vi "Constructor.vi"(8 "error in (no error)":errorcluster, 11 "Module Settings":T1) -> (0 "error out":errorcluster, 2 "Use?":bool, 3 "Module.lvclass":refnum<class "Module.lvclass">)   [LabVIEW 2025, in "Module.lvclass"]
doc: "Instantiate specific module class with configured signals."
uses:
  Module.lvclass
  Module Settings.ctl
  Signal/Signal/Signal Settings.ctl
  Input Module/Input Module.lvclass
  C:/Projects/VeriStand-FPGA-Generation-Wizard/Source/Classes/Module/Module/Module.lvclass
  Output Module/Output Module.lvclass
  VI/VI/Error Codes.ctl
  Module.lvclass/Module.ctl
  Signal/Signal/Signal.lvclass
  VI/VI/VI.lvclass
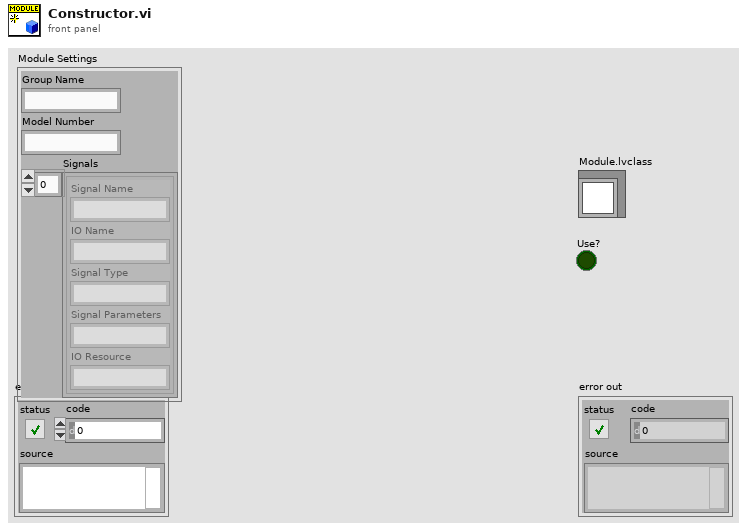
[diagram p1: front panel]
types:
  T1 = typedef "Module.lvclass/Module Settings.ctl" = cluster{"Group Name":string, "Model Number":string, "Signals":T2[]}
  T2 = typedef "Signal.lvclass/Signal Settings.ctl" = cluster{"Signal Name":string, "IO Name":string, "Signal Type":string, "Signal Parameters":string, "IO Resource":string}
  T3 = typedef "VI.lvclass/Error Codes.ctl" = enum16{"Signal Unsupported", "Module Unsupported", "Parameter Unsupported", "Signal Code Gen Error", "Module Code Gen Error", "Cleanup Code Error", "Signal Direction Mismatch", "Signal Type Mismatch", "Module Channel Number Mismatch", "Minimum Channels Mismatch"}
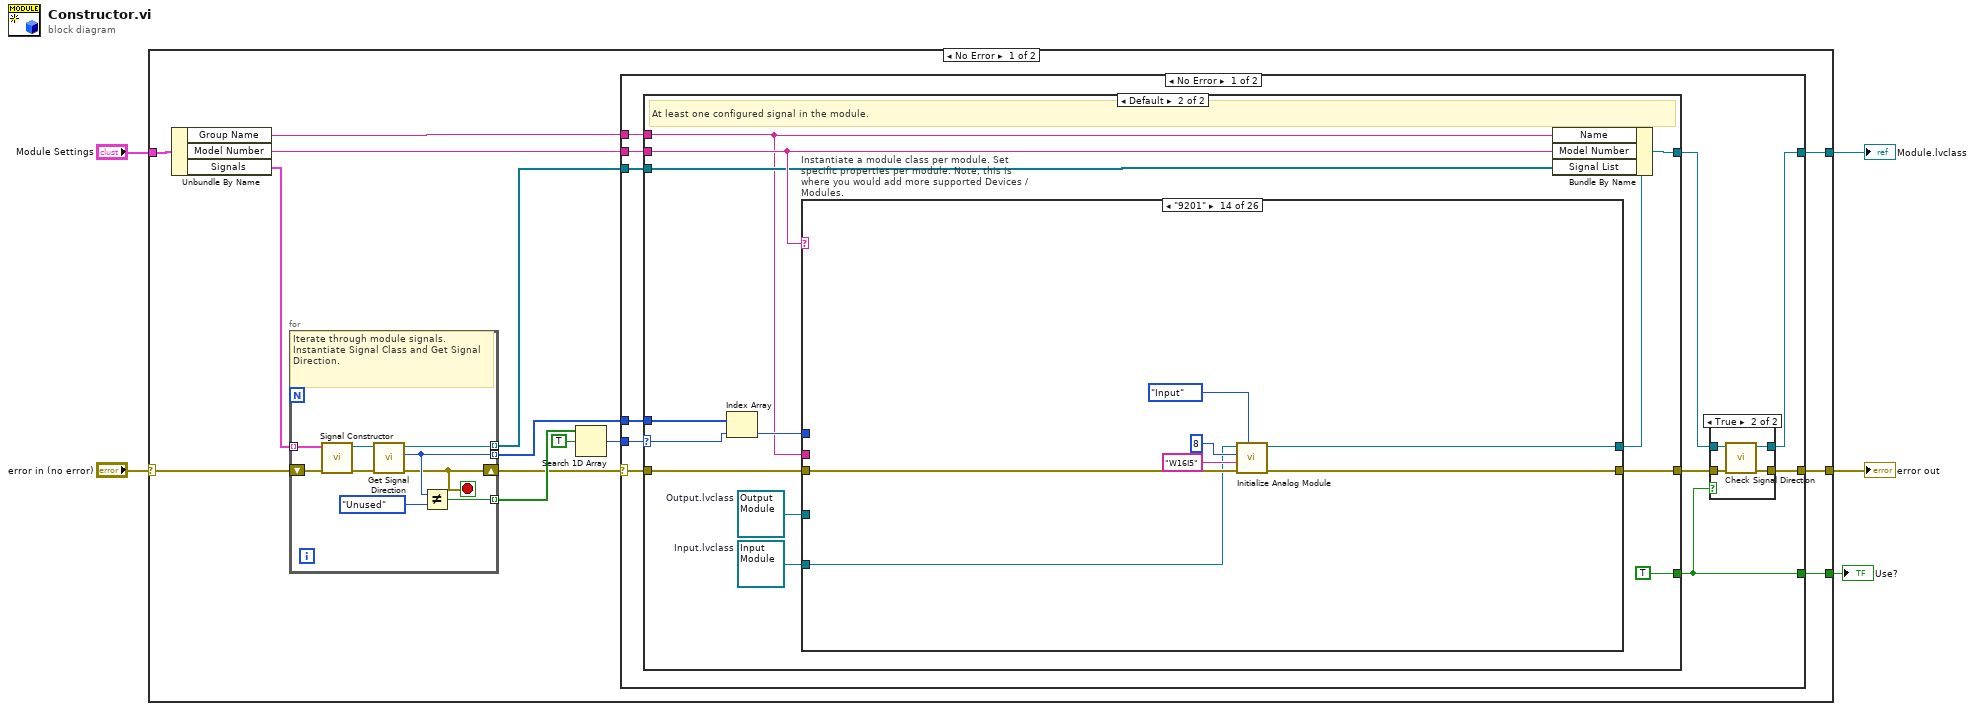
[diagram p0: block diagram]
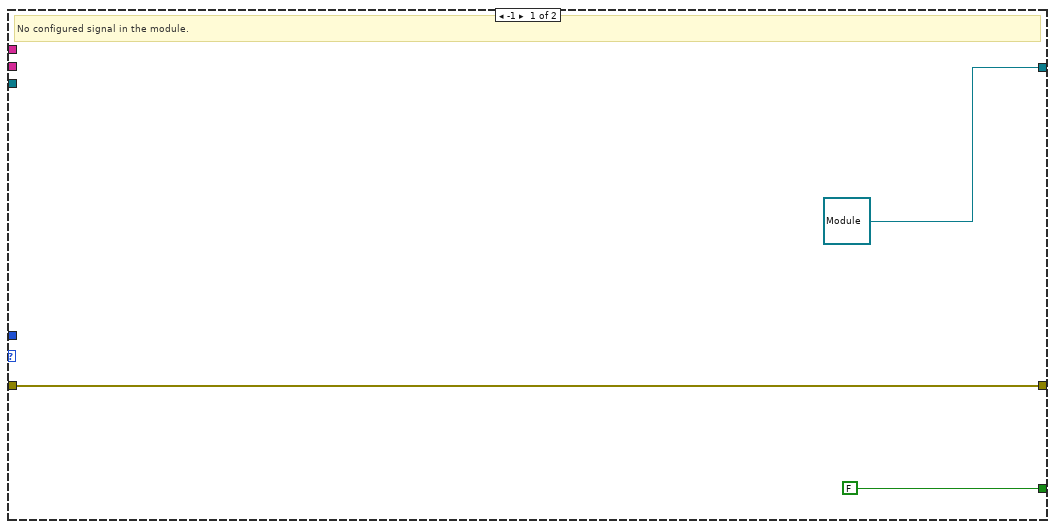
[diagram p3: hidden frame]
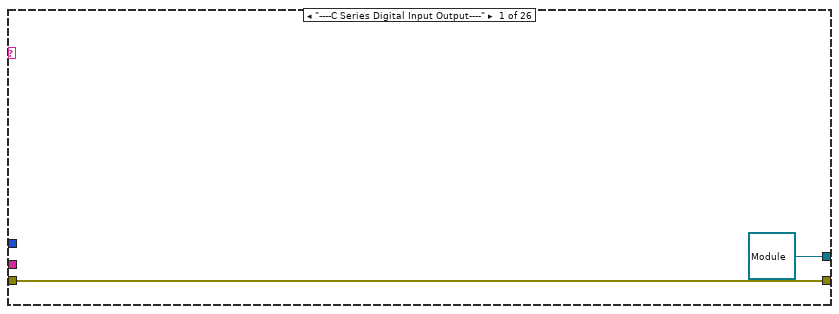
[diagram p4: hidden frame]
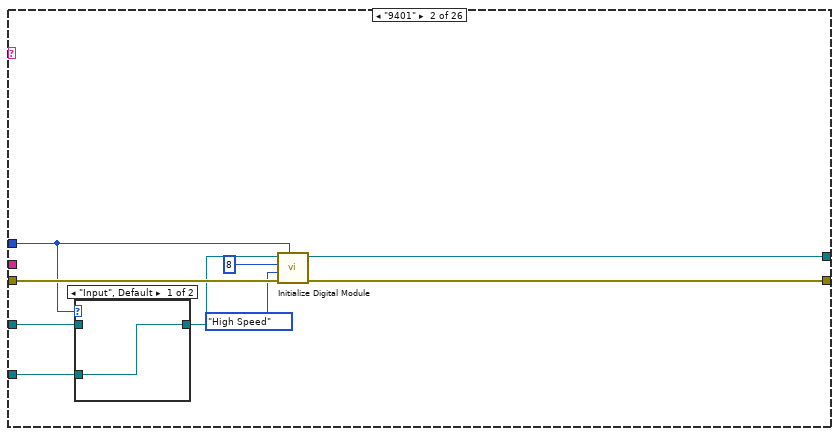
[diagram p5: hidden frame]
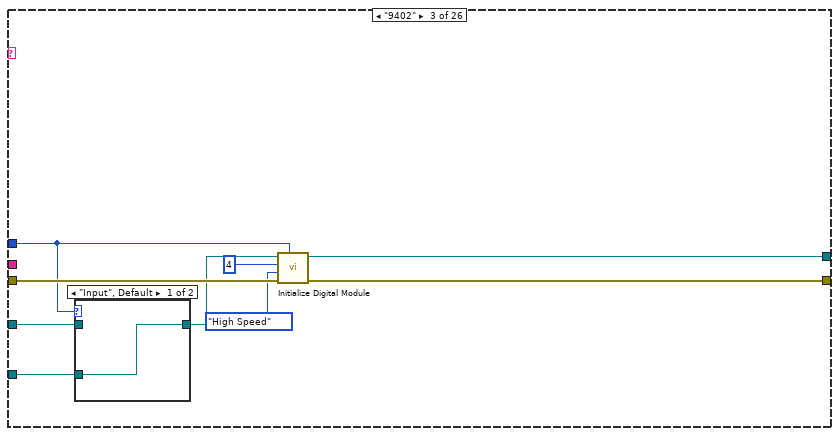
[diagram p7: hidden frame]
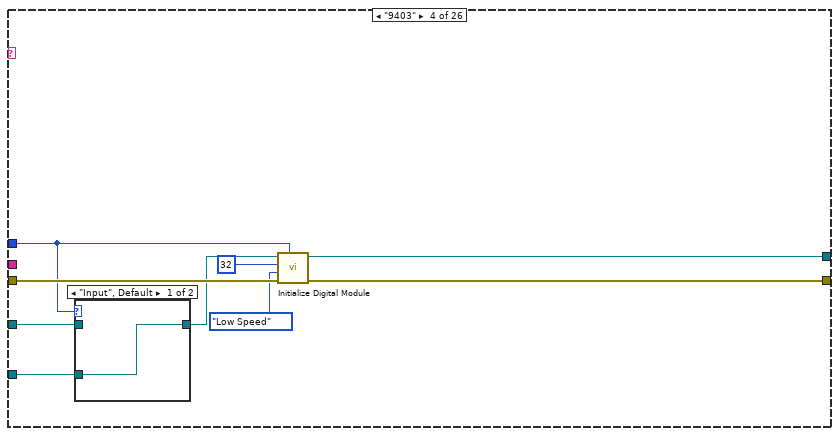
[diagram p9: hidden frame]
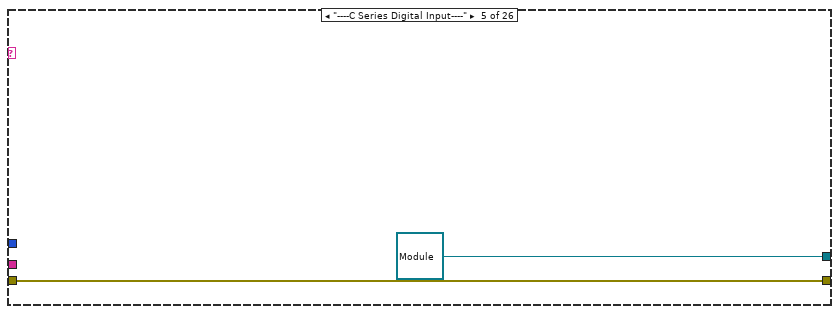
[diagram p11: hidden frame]
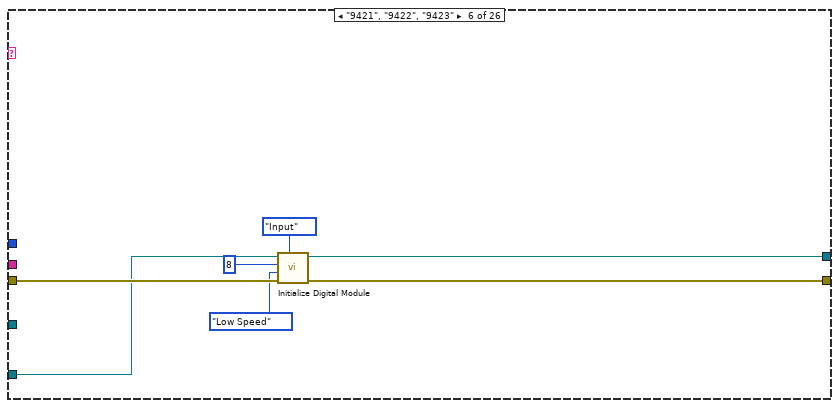
[diagram p12: hidden frame]
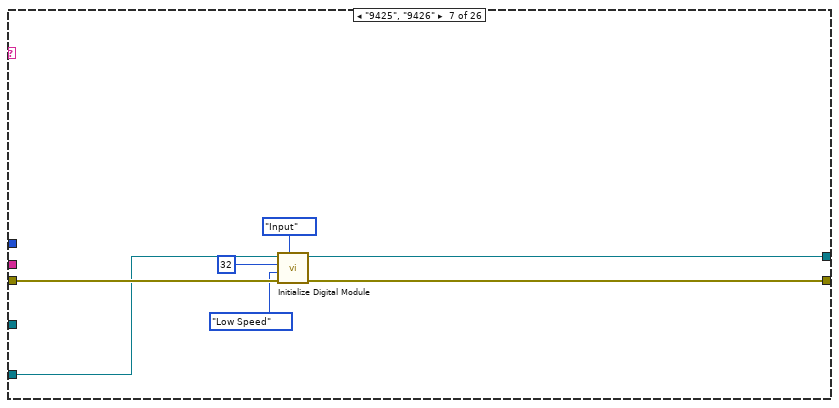
[diagram p13: hidden frame]
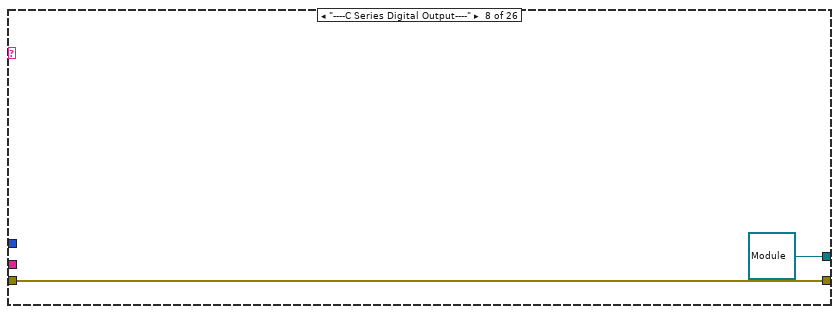
[diagram p14: hidden frame]
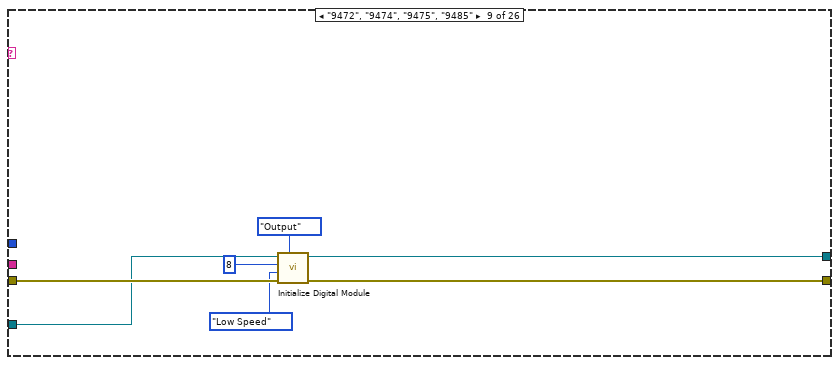
[diagram p15: hidden frame]
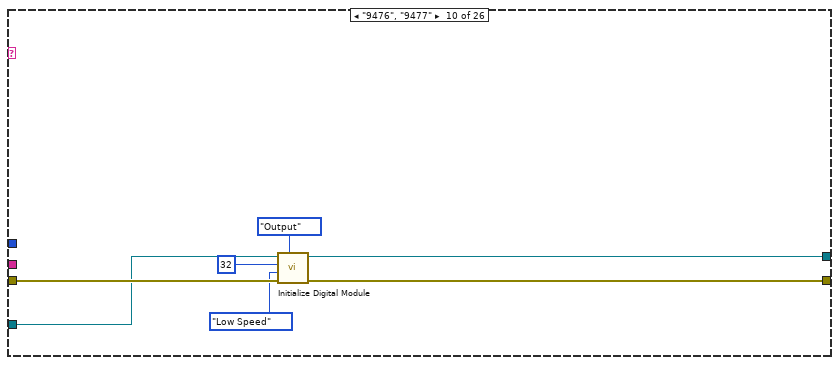
[diagram p16: hidden frame]
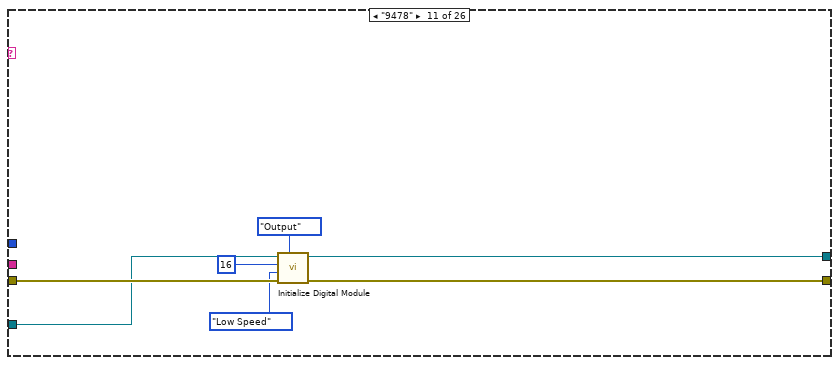
[diagram p17: hidden frame]
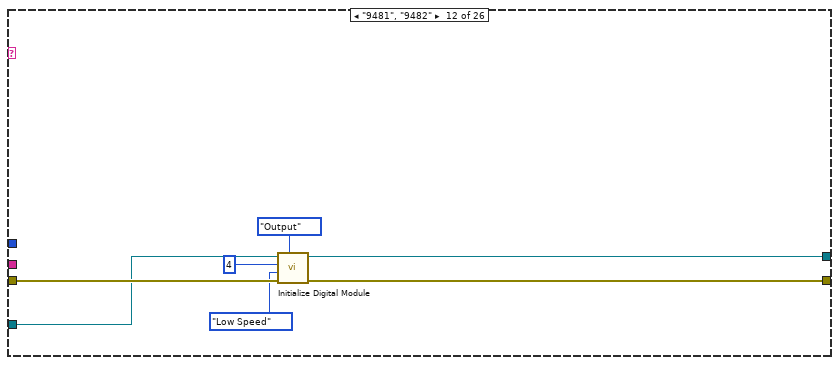
[diagram p18: hidden frame]
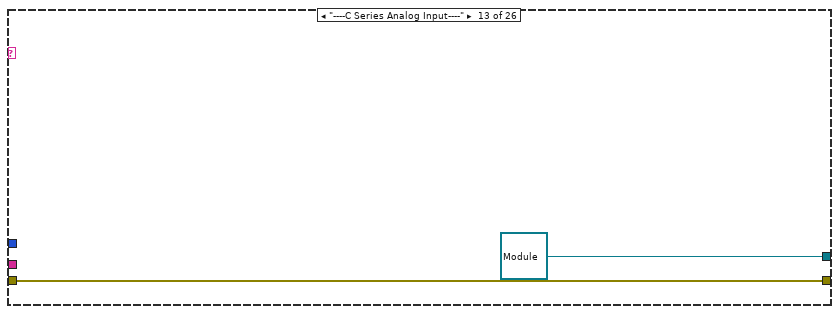
[diagram p19: hidden frame]
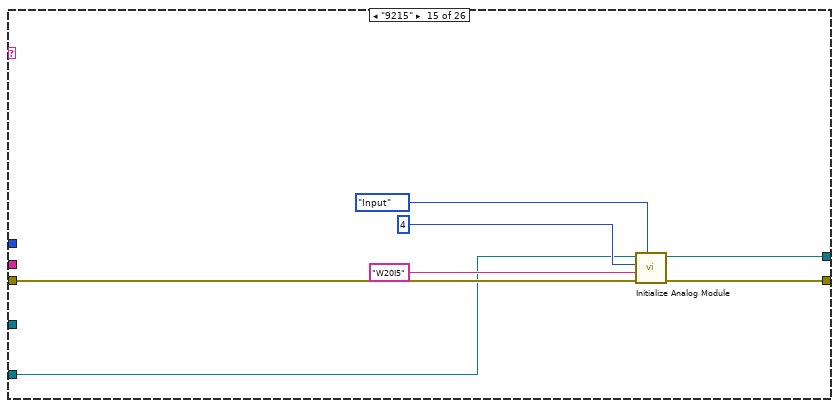
[diagram p20: hidden frame]
diagram:
  n1 = case shown="No Error" "error in (no error)" {
    selector: "error in (no error)" -> [w13 w285]
    tunnel: "Module Settings" -> [w19 _]
    tunnel: [w18 refnum<class "Module.lvclass"> refnum ("Module out")] -> w4
    tunnel: [w15 w285] -> w2
    tunnel: [w7 FALSE] -> w1
    frame No Error {
      n2 = Unbundle By Name(w19) -> ("Group Name"=w17:string, "Model Number"=w16:string, "Signals"=w14:T2[])
      n3 = for {
        tunnel: w14 -> [w282] mode=indexing
        shift-right: [w274] -> w6
        shift-left: w13 -> [w281]
        tunnel: [w278] -> w12 mode=indexing
        tunnel: [w277] -> w9 mode=indexing
        tunnel: [w275] -> w11 mode=indexing
        stop <- w274 stop-if-true
        # "Iterate through module signals. Instantiate Signal Class and Get Signal Direction."
        n4 = call "Signal Constructor.vi"("error in (no error)"=w281, "Signal Settings"=w282) -> ("error out"=w280:errorcluster, "IO Class.lvclass"=w279:refnum<class "Signal.lvclass">)  [unwired: 8 in]
        n5 = call "Get Signal Direction.vi"("error in (no error)"=w280, "IO Class in"=w279) -> ("error out"=w274:errorcluster, "Direction"=w277:enum16{"Input", "Output", "Unused"}, "IO Class out"=w278:refnum<class "Signal.lvclass">)  [unwired: 7 in]
        n6 = Not Equal?(x=w277, y=enum16{"Input", "Output", "Unused"}."Unused" ("Direction")) -> (x != y?=w275:bool)
      }
      n7 = Search 1D Array(1D array=w11, element=TRUE) -> (index of element=w8:i32)  [unwired: 1 in]
      n8 = case shown="No Error" w6 {
        selector: w6 -> [w25 w273]
        tunnel: [w21 refnum<class "Module.lvclass"> refnum ("Module out")] -> w18
        tunnel: w17 -> [w30 _]
        tunnel: w16 -> [w29 _]
        tunnel: [w23 w273] -> w15
        tunnel: w12 -> [w28 _]
        tunnel: w9 -> [w27 _]
        tunnel: w8 -> [w26 _]
        tunnel: [w20 _] -> w7
        frame No Error {
          n9 = case shown="Default" w26 {
            selector: w26 -> [_ w42]
            tunnel: [refnum<class "Module.lvclass"> refnum ("Module out") w51] -> w22
            tunnel: w30 -> [_ w40]
            tunnel: w29 -> [_ w50]
            tunnel: [w39 w49] -> w24
            tunnel: w28 -> [_ w46]
            tunnel: w25 -> [w39 w45]
            tunnel: w27 -> [_ w44]
            tunnel: [FALSE TRUE] -> w20
            frame -1 {
              # "No configured signal in the module."
            }
            frame Default {
              w47 = refnum<class "Output Module.lvclass"> refnum  # Output.lvclass
              w48 = refnum<class "Input Module.lvclass"> refnum  # Input.lvclass
              # "At least one configured signal in the module."
              n10 = Index Array(array=w44, index=w42) -> (element=w43:enum16{"Input", "Output", "Unused"})
              n11 = case "Instantiate a module class per module. Set specific properties per module. Note, this is where you would add more supported Devices / Modules." shown="\"9201\"" w50 {
                selector: w50 -> [_ _ _ _ _ _ _ _ _ _ _ _ _ _ _ _ _ _ _ _ _ _ _ _ _ w210]
                tunnel: [refnum<class "Module.lvclass"> refnum ("Module out") w63 w74 w85 refnum<class "Module.lvclass"> refnum ("Module out") w96 w103 refnum<class "Module.lvclass"> refnum ("Module out") w112 w119 w126 w133 refnum<class "Module.lvclass"> refnum ("Module out") w142 w149 w156 w163 w170 w177 w184 refnum<class "Module.lvclass"> refnum ("Module out") w193 w200 w207 refnum<class "Module.lvclass"> refnum ("Module out") w216] -> w52
                tunnel: w45 -> [w54 w62 w73 w84 w89 w95 w102 w105 w111 w118 w125 w132 w135 w137 w144 w151 w158 w165 w172 w179 w186 w192 w199 w206 w209 w220]
                tunnel: [w54 w61 w72 w83 w89 w94 w101 w105 w110 w117 w124 w131 w135 w141 w148 w155 w162 w169 w176 w183 w186 w191 w198 w205 w209 w215] -> w49
                tunnel: w43 -> [_ w58 w69 w80 _ _ _ _ _ _ _ _ _ _ _ _ _ _ _ _ _ _ _ _ _ w217]
                tunnel: w48 -> [_ w56 w67 w78 _ w91 w98 _ _ _ _ _ _ w136 w143 w150 w157 w164 w171 w178 _ _ _ _ _ w218]
                tunnel: w47 -> [_ w57 w68 w79 _ _ _ _ w106 w113 w120 w127 _ _ _ _ _ _ _ _ _ w187 w194 w201 _ w219]
                tunnel: w40 -> [_ _ _ _ _ _ _ _ _ _ _ _ _ _ _ _ _ _ _ _ _ _ _ _ _ w221]
                frame "----C Series Digital Input Output----" {
                }
                frame "9401" {
                  n12 = case shown="\"Input\", Default" w58 {
                    tunnel: w57 -> [_ w65]
                    tunnel: w56 -> [w64 _]
                    tunnel: [w64 w65] -> w55
                    frame "Input", Default {
                    }
                    frame "Output" {
                    }
                  }
                  n13 = call "Initialize Digital Module.vi"("Direction"=w58, "error in (no error)"=w62, "Speed"=enum16{"High Speed", "Low Speed"}."High Speed", "Channels"=u8 8, "Module in"=w55) -> ("error out"=w61:errorcluster, "Module out"=w63:refnum<class "Module.lvclass">)  [unwired: 5 in]
                }
                frame "9402" {
                  n14 = case shown="\"Input\", Default" w69 {
                    tunnel: w68 -> [_ w76]
                    tunnel: w67 -> [w75 _]
                    tunnel: [w75 w76] -> w66
                    frame "Input", Default {
                    }
                    frame "Output" {
                    }
                  }
                  n15 = call "Initialize Digital Module.vi"("Direction"=w69, "error in (no error)"=w73, "Speed"=enum16{"High Speed", "Low Speed"}."High Speed", "Channels"=u8 4, "Module in"=w66) -> ("error out"=w72:errorcluster, "Module out"=w74:refnum<class "Module.lvclass">)  [unwired: 5 in]
                }
                frame "9403" {
                  n16 = case shown="\"Input\", Default" w80 {
                    tunnel: w79 -> [_ w87]
                    tunnel: w78 -> [w86 _]
                    tunnel: [w86 w87] -> w77
                    frame "Input", Default {
                    }
                    frame "Output" {
                    }
                  }
                  n17 = call "Initialize Digital Module.vi"("Direction"=w80, "error in (no error)"=w84, "Speed"=enum16{"High Speed", "Low Speed"}."Low Speed", "Channels"=u8 32, "Module in"=w77) -> ("error out"=w83:errorcluster, "Module out"=w85:refnum<class "Module.lvclass">)  [unwired: 5 in]
                }
                frame "----C Series Digital Input----" {
                }
                frame "9421", "9422", "9423" {
                  n18 = call "Initialize Digital Module.vi"("Direction"=enum16{"Input", "Output"}."Input", "error in (no error)"=w95, "Speed"=enum16{"High Speed", "Low Speed"}."Low Speed", "Channels"=u8 8, "Module in"=w91) -> ("error out"=w94:errorcluster, "Module out"=w96:refnum<class "Input Module.lvclass">)  [unwired: 5 in]
                }
                frame "9425", "9426" {
                  n19 = call "Initialize Digital Module.vi"("Direction"=enum16{"Input", "Output"}."Input", "error in (no error)"=w102, "Speed"=enum16{"High Speed", "Low Speed"}."Low Speed", "Channels"=u8 32, "Module in"=w98) -> ("error out"=w101:errorcluster, "Module out"=w103:refnum<class "Input Module.lvclass">)  [unwired: 5 in]
                }
                frame "----C Series Digital Output----" {
                }
                frame "9472", "9474", "9475", "9485" {
                  n20 = call "Initialize Digital Module.vi"("Direction"=enum16{"Input", "Output"}."Output", "error in (no error)"=w111, "Speed"=enum16{"High Speed", "Low Speed"}."Low Speed", "Channels"=u8 8, "Module in"=w106) -> ("error out"=w110:errorcluster, "Module out"=w112:refnum<class "Output Module.lvclass">)  [unwired: 5 in]
                }
                frame "9476", "9477" {
                  n21 = call "Initialize Digital Module.vi"("Direction"=enum16{"Input", "Output"}."Output", "error in (no error)"=w118, "Speed"=enum16{"High Speed", "Low Speed"}."Low Speed", "Channels"=u8 32, "Module in"=w113) -> ("error out"=w117:errorcluster, "Module out"=w119:refnum<class "Output Module.lvclass">)  [unwired: 5 in]
                }
                frame "9478" {
                  n22 = call "Initialize Digital Module.vi"("Direction"=enum16{"Input", "Output"}."Output", "error in (no error)"=w125, "Speed"=enum16{"High Speed", "Low Speed"}."Low Speed", "Channels"=u8 16, "Module in"=w120) -> ("error out"=w124:errorcluster, "Module out"=w126:refnum<class "Output Module.lvclass">)  [unwired: 5 in]
                }
                frame "9481", "9482" {
                  n23 = call "Initialize Digital Module.vi"("Direction"=enum16{"Input", "Output"}."Output", "error in (no error)"=w132, "Speed"=enum16{"High Speed", "Low Speed"}."Low Speed", "Channels"=u8 4, "Module in"=w127) -> ("error out"=w131:errorcluster, "Module out"=w133:refnum<class "Output Module.lvclass">)  [unwired: 5 in]
                }
                frame "----C Series Analog Input----" {
                }
                frame "9201" {
                  n24 = call "Initialize Analog Module.vi"("Direction"=enum16{"Input", "Output"}."Input", "error in (no error)"=w137, "FXP Type"="W16I5", "Channels"=u8 8, "Module in"=w136) -> ("error out"=w141:errorcluster, "Module out"=w142:refnum<class "Input Module.lvclass">)  [unwired: 5 in]
                }
                frame "9215" {
                  n25 = call "Initialize Analog Module.vi"("Direction"=enum16{"Input", "Output"}."Input", "error in (no error)"=w144, "FXP Type"="W20I5", "Channels"=u8 4, "Module in"=w143) -> ("error out"=w148:errorcluster, "Module out"=w149:refnum<class "Input Module.lvclass">)  [unwired: 5 in]
                }
                frame "9220" {
                  n26 = call "Initialize Analog Module.vi"("Direction"=enum16{"Input", "Output"}."Input", "error in (no error)"=w151, "FXP Type"="W24I5", "Channels"=u8 16, "Module in"=w150) -> ("error out"=w155:errorcluster, "Module out"=w156:refnum<class "Input Module.lvclass">)  [unwired: 5 in]
                }
                frame "9221" {
                  n27 = call "Initialize Analog Module.vi"("Direction"=enum16{"Input", "Output"}."Input", "error in (no error)"=w158, "FXP Type"="W16I7", "Channels"=u8 8, "Module in"=w157) -> ("error out"=w162:errorcluster, "Module out"=w163:refnum<class "Input Module.lvclass">)  [unwired: 5 in]
                }
                frame "9222", "9223" {
                  n28 = call "Initialize Analog Module.vi"("Direction"=enum16{"Input", "Output"}."Input", "error in (no error)"=w165, "FXP Type"="W24I5", "Channels"=u8 4, "Module in"=w164) -> ("error out"=w169:errorcluster, "Module out"=w170:refnum<class "Input Module.lvclass">)  [unwired: 5 in]
                }
                frame "9224" {
                  n29 = call "Initialize Analog Module.vi"("Direction"=enum16{"Input", "Output"}."Input", "error in (no error)"=w172, "FXP Type"="W24I5", "Channels"=u8 8, "Module in"=w171) -> ("error out"=w176:errorcluster, "Module out"=w177:refnum<class "Input Module.lvclass">)  [unwired: 5 in]
                }
                frame "9228" {
                  n30 = call "Initialize Analog Module.vi"("Direction"=enum16{"Input", "Output"}."Input", "error in (no error)"=w179, "FXP Type"="W24I7", "Channels"=u8 8, "Module in"=w178) -> ("error out"=w183:errorcluster, "Module out"=w184:refnum<class "Input Module.lvclass">)  [unwired: 5 in]
                }
                frame "----C Series Analog Output----" {
                }
                frame "9262" {
                  n31 = call "Initialize Analog Module.vi"("Direction"=enum16{"Input", "Output"}."Output", "error in (no error)"=w192, "FXP Type"="W20I5", "Channels"=u8 6, "Module in"=w187) -> ("error out"=w191:errorcluster, "Module out"=w193:refnum<class "Output Module.lvclass">)  [unwired: 5 in]
                }
                frame "9263", "9269" {
                  n32 = call "Initialize Analog Module.vi"("Direction"=enum16{"Input", "Output"}."Output", "error in (no error)"=w199, "FXP Type"="W20I5", "Channels"=u8 4, "Module in"=w194) -> ("error out"=w198:errorcluster, "Module out"=w200:refnum<class "Output Module.lvclass">)  [unwired: 5 in]
                }
                frame "9264" {
                  n33 = call "Initialize Analog Module.vi"("Direction"=enum16{"Input", "Output"}."Output", "error in (no error)"=w206, "FXP Type"="W20I5", "Channels"=u8 16, "Module in"=w201) -> ("error out"=w205:errorcluster, "Module out"=w207:refnum<class "Output Module.lvclass">)  [unwired: 5 in]
                }
                frame "----R Series----" {
                }
                frame Default {
                  # "Assume R Series"
                  n34 = Match Pattern(string=w210, regular expression="-") -> (after substring=w213:string)  [unwired: 1 in, 3 out]
                  n35 = Search 1D Array(1D array=string[] ["7811R", "7813R", "7830R", "7831R", "7833R", "7820R", "7821R", "7822R", "7845R", "7846R", "7847R", "7855R", "7856R", "7857R", "7858R", "7861R", "7862R"], element=w213) -> (index of element=w211:i32)  [unwired: 1 in]
                  n36 = case shown="-1" w211 {
                    tunnel: w221 -> [w223 w228]
                    tunnel: w220 -> [w226 w235]
                    tunnel: w219 -> [_ w234]
                    tunnel: w218 -> [_ w233]
                    tunnel: w217 -> [_ w232]
                    tunnel: [refnum<class "Module.lvclass"> refnum ("Module out") w231] -> w216
                    tunnel: [w225 w230] -> w215
                    tunnel: w210 -> [w224 w229]
                    frame -1 {
                      # "Not R Series or not supported"
                      n37 = call "Error Codes.vi"("Error"=Error_Codes."Module Unsupported", "error in (no error)"=w226, "Module/Signal Name"=w223, "Module/Signal Resource"=w224) -> ("error out"=w225:errorcluster)  [unwired: 7 in]
                    }
                    frame Default {
                      # "Supported R Series"
                      n38 = call <vilib>:"Space Constant.vi"() -> ("String"=w239:string)
                      n39 = Spreadsheet String To Array(delimiter (Tab)=w239, format string="%s", spreadsheet string=w228, array type (2D Dbl)=string[] []) -> (array=w238:string[])
                      n40 = Index Array(array=w238) -> (element #2=w236:string)  [unwired: 2 in, 1 out]
                      n41 = case shown="Default" w236 {
                        tunnel: w235 -> [w244 w251 w261 w270]
                        tunnel: w234 -> [_ w248 w260 _]
                        tunnel: w233 -> [w243 _ w259 _]
                        tunnel: w232 -> [_ _ w255 _]
                        tunnel: [w241 w249 w257 refnum<class "Module.lvclass"> refnum ("Module out")] -> w231
                        tunnel: [w242 w250 w256 w269] -> w230
                        tunnel: w229 -> [_ _ _ w267]
                        tunnel: w228 -> [_ _ _ w266]
                        frame "AI" {
                          n42 = call "Initialize Analog Module.vi"("Direction"=enum16{"Input", "Output"}."Input", "error in (no error)"=w244, "FXP Type"="W27I5", "Channels"=u8 8, "Module in"=w243) -> ("error out"=w242:errorcluster, "Module out"=w241:refnum<class "Input Module.lvclass">)  [unwired: 5 in]
                        }
                        frame "AO" {
                          n43 = call "Initialize Analog Module.vi"("Direction"=enum16{"Input", "Output"}."Output", "error in (no error)"=w251, "FXP Type"="W20I5", "Channels"=u8 8, "Module in"=w248) -> ("error out"=w250:errorcluster, "Module out"=w249:refnum<class "Output Module.lvclass">)  [unwired: 5 in]
                        }
                        frame "DIO" {
                          n44 = case shown="\"Input\", Default" w255 {
                            tunnel: w260 -> [_ w265]
                            tunnel: w259 -> [w264 _]
                            tunnel: [w264 w265] -> w258
                            frame "Input", Default {
                            }
                            frame "Output" {
                            }
                          }
                          n45 = call "Initialize Digital Module.vi"("Direction"=w255, "error in (no error)"=w261, "Speed"=enum16{"High Speed", "Low Speed"}."High Speed", "Channels"=u8 8, "Module in"=w258) -> ("error out"=w256:errorcluster, "Module out"=w257:refnum<class "Module.lvclass">)  [unwired: 5 in]
                        }
                        frame Default {
                          n46 = call "Error Codes.vi"("Error"=Error_Codes."Module Unsupported", "error in (no error)"=w270, "Module/Signal Name"=w266, "Module/Signal Resource"=w267) -> ("error out"=w269:errorcluster)  [unwired: 7 in]
                        }
                      }
                    }
                  }
                }
              }
              n47 = Bundle By Name(cluster=w52, "Name"=w40, "Model Number"=w50, "Signal List"=w46) -> (w51:refnum<class "Module.lvclass">)
            }
          }
          n48 = case shown="True" w20 {
            tunnel: w24 -> [w32 w36]
            tunnel: [w32 w35] -> w23
            tunnel: w22 -> [w31 w34]
            tunnel: [w31 w33] -> w21
            frame False {
            }
            frame True {
              n49 = call "Check Signal Direction.vi"("error in (no error)"=w36, "Module in"=w34) -> ("error out"=w35:errorcluster, "Module out"=w33:refnum<class "Module.lvclass">)  [unwired: 8 in]
            }
          }
        }
        frame Error {
        }
      }
    }
    frame Error {
    }
  }
  "Module.lvclass" <- w4
  "error out" <- w2
  "Use?" <- w1
